vi "GetWaveformChannelName.vi"(8 "error in (no error)":errorcluster, 11 "waveform in":waveform(sgl)) -> (0 "error out":errorcluster, 2 "name":string, 3 "waveform out":waveform(sgl))   [LabVIEW 2017]
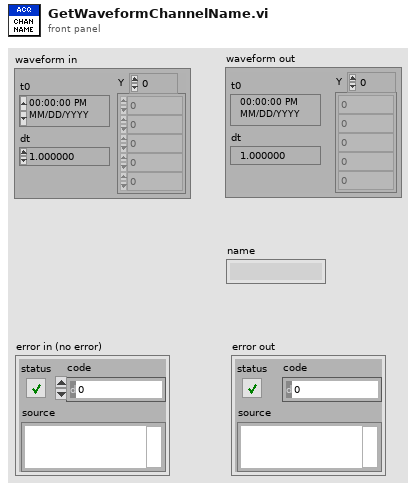
[diagram p1: front panel]
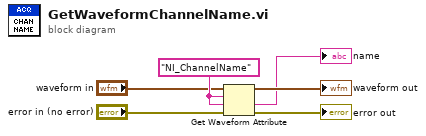
[diagram p0: block diagram]
diagram:
  w5 = "NI_ChannelName" ("name")
  n1 = Get Waveform Attribute(4:"error in (no error)", 5:w5, 6:w5, 7:"waveform in") -> (0:→"error out":errorcluster, 1:→"name":string, 3:→"waveform out":waveform(sgl))  [unwired: 1 out]
